vi "HW_Configuration.LoadDevice.vi"(8 "error in":errorcluster, 9 "name":string, 10 "XML file path":path=path "C:/Projects/TM-OS/trunk/Design/XML_HW_config2.xml", 11 "cluster in":refnum<vi>) -> (0 "error out":errorcluster, 2 "config":variant)   [LabVIEW 2019, in "Tools.lvlib"]
uses:
  Tools.lvlib
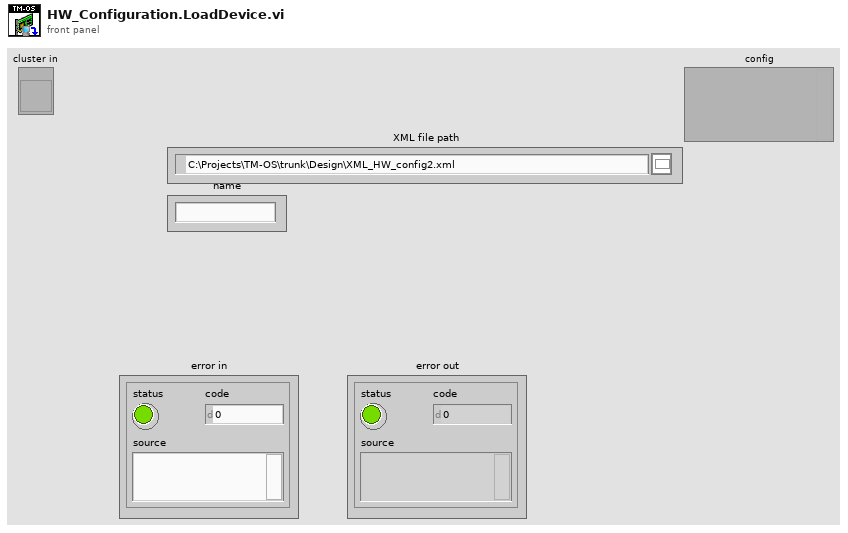
[diagram p1: front panel]
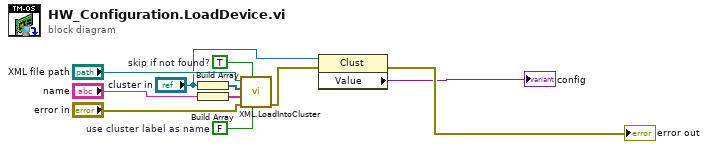
[diagram p0: block diagram]
diagram:
  w6 = FALSE  # use cluster label as name
  w7 = TRUE  # skip if not found?
  n1 = Build Array("cluster in") -> (w11:refnum<vi>[])
  n2 = Build Array("name") -> (w1:string[])
  n3 = call "XML.LoadIntoCluster.vi"("use cluster label as name"=w6, "skip if not found?"=w7, "error in"="error in", "name"=w1, "clusters refs"=w11, "XML file path"="XML file path") -> ("error out"=w4:errorcluster)  [unwired: 5 in]
  n4 = property class="Clust"(reference="cluster in", error in=w4) -> (error out=→"error out":errorcluster, "Value"=→"config":variant)  [unwired: 1 out]
